vi "make_video.vi"() -> ()   [LabVIEW 2011]
panel:
  out "x-y":dbl
  in  "AVI Path":path
  out "Image Out":T1(plugin-control)
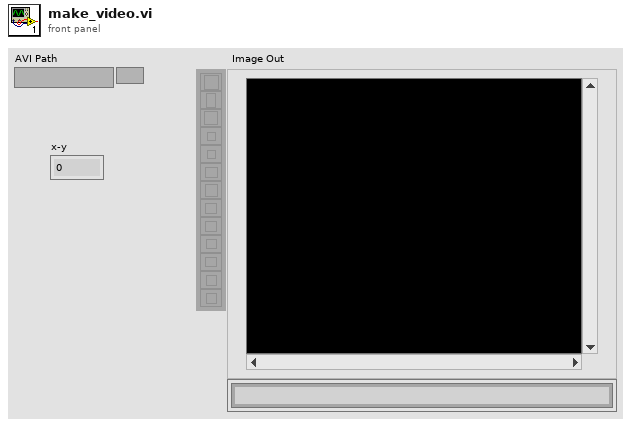
[diagram p1: front panel]
types:
  T1 = typedef "IMAQ Image.ctl" = refnum<image>
  T2 = typedef "AviRefnum.ctl" = refnum<k1>
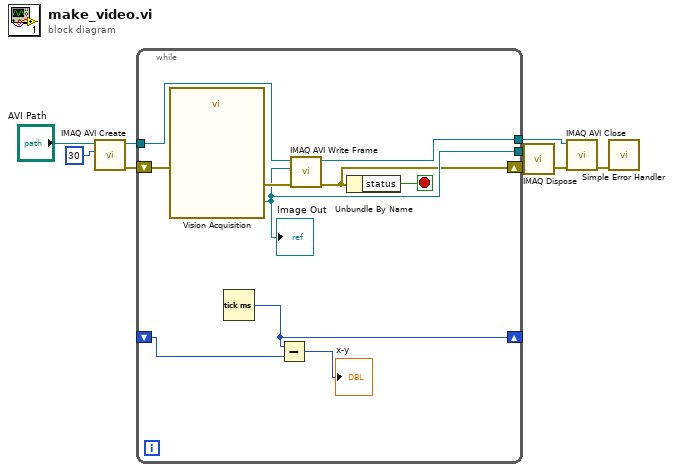
[diagram p0: block diagram]
diagram:
  n1 = call "IMAQ AVI Create"("Frames Per Second"=u32 30, "AVI Path"="AVI Path") -> ("error out"=w9:errorcluster, "Avi Refnum"=w8:T2)  [unwired: 8 in]
  n2 = while {
    shift-right: [w14] -> w7
    shift-left: w9 -> [w19]
    tunnel: w8 -> [w18]
    tunnel: [w16] -> w6
    tunnel: [w15] -> w4
    shift-right: [w12] -> _
    shift-left: _ -> [w10]
    stop <- w13 stop-if-true
    n3 = call "Vision Acquisition"("error in"=w19) -> ("Image Out"=w16:T1, "error out"=w17:errorcluster)  [unwired: 25 in]
    "Image Out" <- w16
    n4 = Tick Count (ms)() -> (millisecond timer value=w12:u32)
    n5 = Subtract(x=w12, y=w10) -> (x-y=→"x-y":u32)
    n6 = call "IMAQ AVI Write Frame"("error in (no error)"=w17, "Image"=w16, "Avi Refnum"=w18) -> ("error out"=w14:errorcluster, "Avi Refnum (duplicate)"=w15:T2)  [unwired: 7 in]
    n7 = Unbundle By Name(w14) -> ("status"=w13:bool)
  }
  n8 = call "IMAQ Dispose"("Image"=w6, "error in (no error)"=w7) -> ("error out"=w5:errorcluster)  [unwired: 4 in]
  n9 = call "IMAQ AVI Close"("error in (no error)"=w5, "Avi Refnum"=w4) -> ("error out"=w3:errorcluster)  [unwired: 9 in]
  n10 = call <vilib>:"Simple Error Handler.vi"("error in (no error)"=w3) -> ()  [unwired: 4 in, 5 out]
